vi "positionFPonMouseDown.vi"(8 "error in":errorcluster, 9 "VI Refnum":refnum<vi>, 10 "Button (from Mouse Down event)":u16, 11 "mouse Device ID in":refnum<k1>) -> (0 "error out":errorcluster, 3 "mouse device ID out":refnum<k1>)   [LabVIEW 2018]
doc: "To be used in a Mouse Down event case, this VI will reposition the calling VI's front panel as long as the left mouse button is held down."
uses:
  <vilib>/Utility/inputDevices.llb/mouseAcquire.vi
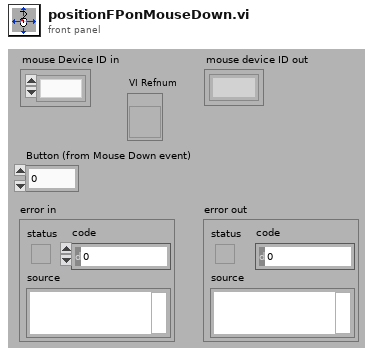
[diagram p1: front panel]
types:
  T1 = typedef "LVRectTypeDef.ctl" = cluster{"Left":i16, "Top":i16, "Right":i16, "Bottom":i16}
  T2 = cluster{"Horizontal":i32, "Vertical":i32, "Scrolling":i32}
  T3 = cluster{"button 1":bool, "button 2":bool, "button 3":bool, "button 4":bool}
  T4 = cluster{"Horizontal":i32, "Vertical":i32, "Horizontal":i32, "Vertical":i32}
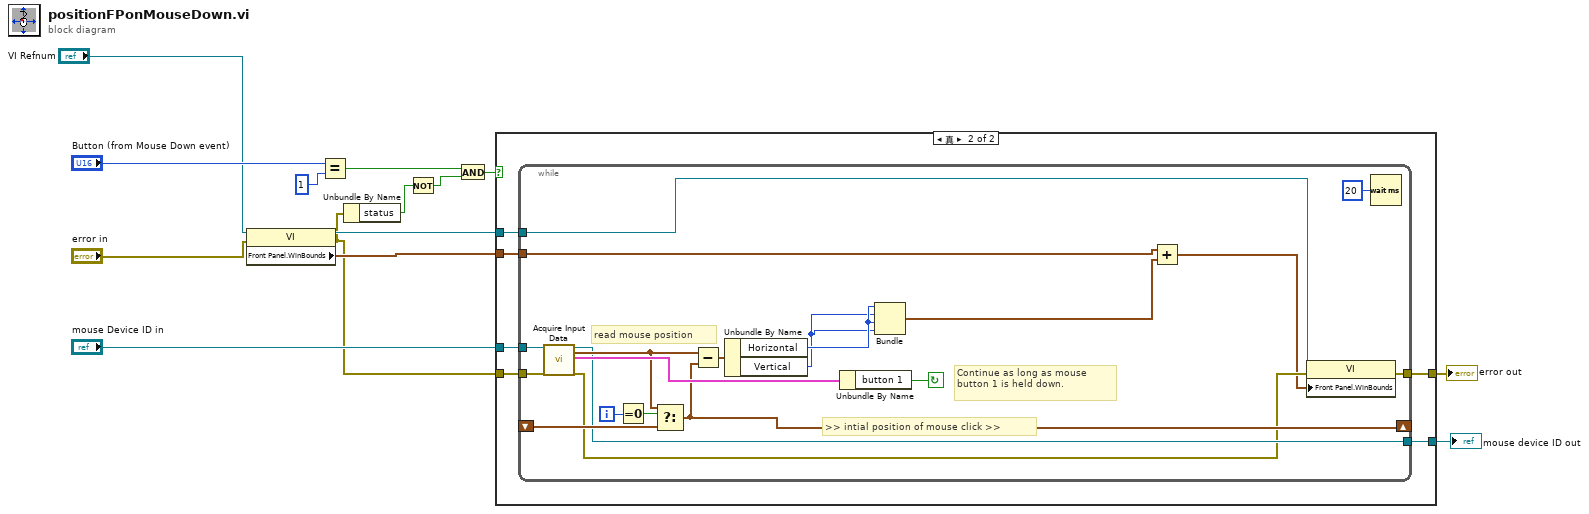
[diagram p0: block diagram]
diagram:
  n1 = property class="VI"(reference="VI Refnum", error in="error in") -> (reference out=w9:refnum<vi>, error out=w4:errorcluster, "Front Panel.WinBounds"=w10:T1)
  n2 = Equal?(x="Button (from Mouse Down event)", y=u16 1) -> (x = y?=w8:bool)
  n3 = Unbundle By Name(w4) -> ("status"=w7:bool)
  n4 = Not(x=w7) -> (.not. x?=w6:bool)
  n5 = And(x=w8, y=w6) -> (x .and. y?=w5:bool)
  n6 = case shown="真" w5 {
    tunnel: "mouse Device ID in" -> [w16 w22]
    tunnel: w10 -> [_ w21]
    tunnel: [w16 w20] -> w14
    tunnel: w9 -> [_ w19]
    tunnel: w4 -> [w15 w18]
    tunnel: [w15 w17] -> w3
    frame False {
      # "Not button 1, or error"
    }
    frame True {
      n7 = while {
        tunnel: w22 -> [w42]
        shift-right: [w34] -> _
        shift-left: _ -> [w39]
        tunnel: w21 -> [w27]
        tunnel: [w32] -> w20
        tunnel: w19 -> [w31]
        tunnel: w18 -> [w30]
        tunnel: [w28] -> w17
        i -> [w41]
        stop <- w36 continue-if-true
        # "read mouse position"
        # "Continue as long as mouse\nbutton 1 is held down."
        # ">> intial position of mouse click >>"
        n8 = call-poly <vilib>:"Acquire Input Data.vi"("device ID"=w42, "error in (no error)"=w30) -> ("device ID"=w32:refnum<k1>, "axis info"=w33:T2, "button info"=w37:T3, "error out"=w29:errorcluster)  [unwired: 14 in]
        n9 = Equal To 0?(x=w41) -> (x = 0?=w40:bool)
        n10 = Select(t=w33, s=w40, f=w39) -> (s? t:f=w34:T2)
        n11 = Subtract(x=w33, y=w34) -> (x-y=w38:T2)
        n12 = Unbundle By Name(w38) -> ("Horizontal"=w26:i32, "Vertical"=w25:i32)
        n13 = Unbundle By Name(w37) -> ("button 1"=w36:bool)
        n14 = Bundle("Horizontal"=w26, "Vertical"=w25, "Horizontal"=w26, "Vertical"=w25) -> (w24:T4)  [unwired: 1 in]
        n15 = Add(x=w27, y=w24) -> (x+y=w23:cluster{i32, i32, i32, i32})
        n16 = property class="VI"(reference=w31, error in=w29, "Front Panel.WinBounds"=w23) -> (error out=w28:errorcluster)  [unwired: 1 out]
        n17 = Wait (ms)(milliseconds to wait=u32 20) -> ()  [unwired: 1 out]
      }
    }
  }
  "mouse device ID out" <- w14
  "error out" <- w3
